vi "Global micro_Devices.vi"() -> ()   [LabVIEW 2014]
panel:
  in  "Current Cube":i32
  out "microfabricating":bool
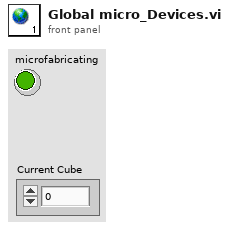
[diagram p1: front panel]
diagram:
